vi "List Principal Things.vi"(8 "error in (no error)":errorcluster, 10 "Principal":string, 11 "IoT Session in":refnum<class "IoT Session.lvclass">) -> (0 "error out":errorcluster, 2 "Principal Things":string[](array[string]), 3 "IoT Session out":refnum<class "IoT Session.lvclass">)   [LabVIEW 2015, in "NI_AWS_IoT.lvlib" / "IoT Session.lvclass"]
uses:
  IoT Session.lvclass
  Core/HTTP Request/Request Options.ctl
  Core/HTTP Request/Name Value Pair.ctl
  Core/HTTP Request/Region handling.ctl
  Core/HTTP Request/URL formatting.ctl
  Core/HTTP Request/HTTP Request.lvclass
  JSON Parsing/NI_JSON Parsing.lvlib
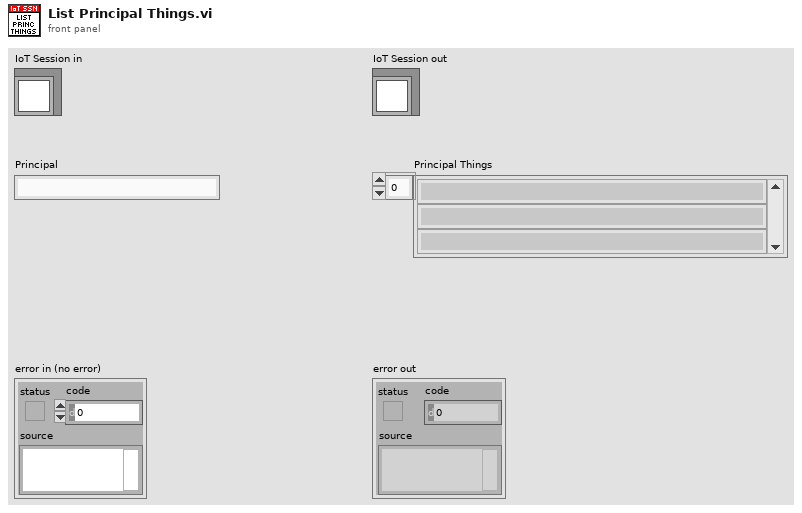
[diagram p1: front panel]
types:
  T1 = typedef "NI_AWS_Core.lvlib/HTTP Request.lvclass/Name Value Pair.ctl" = cluster{"name":string, "value":string}
  T2 = typedef "NI_AWS_Core.lvlib/HTTP Request.lvclass/Request Options.ctl" = cluster{"request headers":T1[], "request parameters":T1[], "request body":string, "region handling":T3, "URL formatting":T4}
  T3 = typedef "NI_AWS_Core.lvlib/HTTP Request.lvclass/Region handling.ctl" = enum16{"use region everywhere", "use region (authentication only)", "use region (URL only)", "ignore region everwhere"}
  T4 = typedef "NI_AWS_Core.lvlib/HTTP Request.lvclass/URL formatting.ctl" = enum16{"region-", "region."}
  T5 = typedef "NI_AWS_Core.lvlib/HTTP Request.lvclass/Response.ctl" = cluster{"Headers":string, "Body":string}
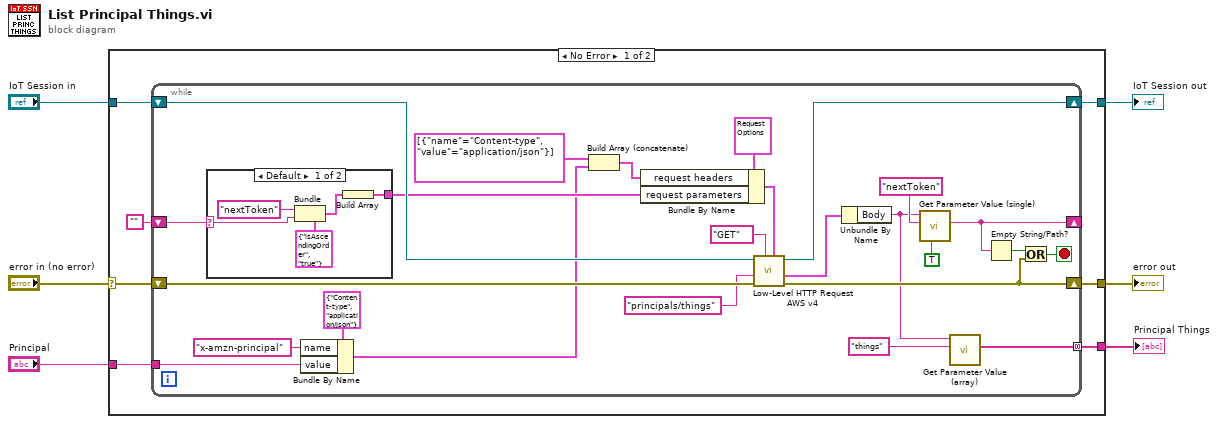
[diagram p0: block diagram]
diagram:
  n1 = case shown="No Error" "error in (no error)" {
    selector: "error in (no error)" -> [w13 w45]
    tunnel: [w12 w45] -> w5
    tunnel: [w11 w44] -> w4
    tunnel: "IoT Session in" -> [w10 w44]
    tunnel: [w8 _] -> w2
    tunnel: "Principal" -> [w7 _]
    frame No Error {
      n2 = while {
        shift-right: [w26] -> w12
        shift-left: w13 -> [w35]
        shift-right: [w34] -> w11
        shift-left: w10 -> [w33]
        shift-right: [w28] -> _
        shift-left: "" -> [w30]
        tunnel: [w14] -> w8 mode=concatenating
        tunnel: w7 -> [w18]
        stop <- w25 stop-if-true
        n3 = case shown="Default" w30 {
          selector: w30 -> [w40 _]
          tunnel: [w43 _] -> w22
          frame Default {
            n4 = Bundle(cluster=T1 {"name"="isAscendingOrder", "value"="true"} ("Name Value Pair"), "name"="nextToken", "value"=w40) -> (w41:T1)
            n5 = Build Array(w41) -> (w43:T1[])
          }
          frame "" {
          }
        }
        n6 = Bundle By Name(cluster=T1 {"name"="Content-type", "value"="application/json"} ("Cluster"), "name"="x-amzn-principal", "value"=w18) -> (w17:T1)
        n7 = Build Array (concatenate)(T1[] [{"name"="Content-type", "value"="application/json"}] ("request headers"), w17) -> (w21:T1[])
        n8 = Bundle By Name(cluster=T2 {"request headers"=[], "request parameters"=[], "request body"="", "region handling"=enum."use region everywhere", "URL formatting"=enum."region."} ("Request Options"), "request headers"=w21, "request parameters"=w22) -> (w36:T2)
        n9 = call "Low-Level HTTP Request AWS v4.vi"("Request Options"=w36, "HTTP-Verb"="GET", "error in (no error)"=w35, "URL Suffix"="principals/things" ("string"), "AWS Core in"=w33) -> ("error out"=w26:errorcluster, "Response"=w31:T5, "AWS Core out"=w34:refnum<class "IoT Session.lvclass">)  [unwired: 3 in, 1 out]
        n10 = Unbundle By Name(w31) -> ("Body"=w16:string)
        n11 = call "Get Parameter Value (single).vi"("Clear Null"=TRUE, "Parameter Name"="nextToken", "JSON"=w16) -> ("Parameter Value"=w28:string)  [unwired: 5 in, 3 out]
        n12 = call "Get Parameter Value (array).vi"("Parameter Name"="things", "JSON"=w16) -> ("Parameter Values"=w14:string[])  [unwired: 7 in, 2 out]
        n13 = Empty String/Path?(string/path=w28) -> (empty?=w27:bool)
        n14 = Or(x=w27, y=w26) -> (x .or. y?=w25:bool)
      }
    }
    frame Error {
    }
  }
  "error out" <- w5
  "IoT Session out" <- w4
  "Principal Things" <- w2
